vi "Indexed String To Enum_csm.vi"(7 "Variant":variant, 8 "error in (no error)":errorcluster, 11 "String":string) -> (0 "error out":errorcluster, 3 "Enum":variant)   [LabVIEW 2017, in "API String Arguments Support.lvlib"]
doc: "Convert String to enum. If string starts with numbers. The conversion is based on number. Otherwise, the conversion is based on the string content. For example: Enum(Spring,Summer,Autumn,Winter). Summer\" could be converted to Enum(Summer). \"1 - anydescription\" could be convert to Enum(Summer) too."
uses:
  API String Arguments Support.lvlib
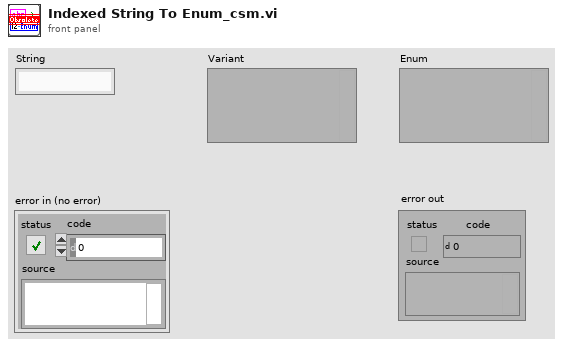
[diagram p1: front panel]
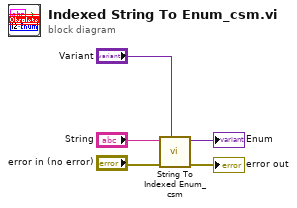
[diagram p0: block diagram]
diagram:
  n1 = call "String To Indexed Enum_csm.vi"("Variant"="Variant", "error in (no error)"="error in (no error)", "String"="String") -> ("error out"=→"error out":errorcluster, "Enum"=→"Enum":variant)  [unwired: 7 in]
